vi "Close Tool Connection.vi"(8 "error in (no error)":errorcluster) -> (0 "error out":errorcluster)   [LabVIEW 2015, in "Tool Interface.lvlib"]
uses:
  Tool Interface.lvlib
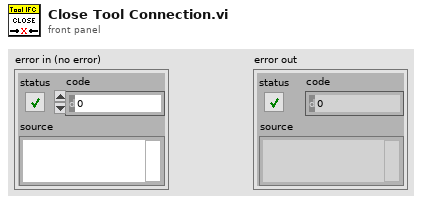
[diagram p1: front panel]
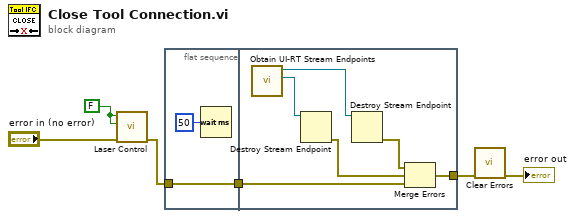
[diagram p0: block diagram]
diagram:
  w6 = FALSE ("Laser 1")
  n1 = call "Laser Control.vi"("error in (no error)"="error in (no error)", "Laser 2"=w6, "Laser 1"=w6) -> ("error out"=w3:errorcluster)  [unwired: 8 in]
  n2 = flat-sequence {
    tunnel: w3 -> [w8]
    tunnel: [w8] -> w2
    tunnel: w2 -> [w10]
    tunnel: [w9] -> w1
    frame #0 {
      n3 = Wait (ms)(milliseconds to wait=u32 50) -> ()  [unwired: 1 out]
    }
    frame #1 {
      n4 = call "Obtain UI-RT Stream Endpoints.vi"() -> ("UI Command Stream"=w11:refnum<k21>, "RT Message Stream"=w12:refnum<k21>)  [unwired: 9 in, 1 out]
      n5 = Destroy Stream Endpoint(11:w11) -> (0:w14:errorcluster)  [unwired: 1 in]
      n6 = Destroy Stream Endpoint(11:w12) -> (0:w13:errorcluster)  [unwired: 1 in]
      n7 = Merge Errors(w13, w14, w10) -> (w9:errorcluster)
    }
  }
  n8 = call <vilib>:"Clear Errors.vi"("error in (no error)"=w1) -> ("error out"=→"error out":errorcluster)  [unwired: 5 in, 1 out]
